vi "Path (SubVI).vi"(1 "File Name":string, 2 "Directory Name":string, 3 "Current VI Name (Case Sensitive)":string, 4 "Current VI Path":path) -> (0 "Path":path)   [LabVIEW 2015]
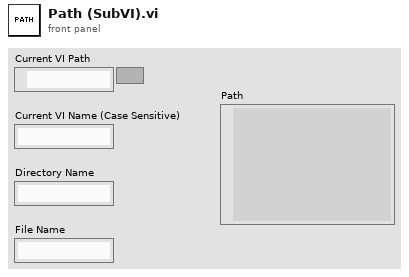
[diagram p1: front panel]
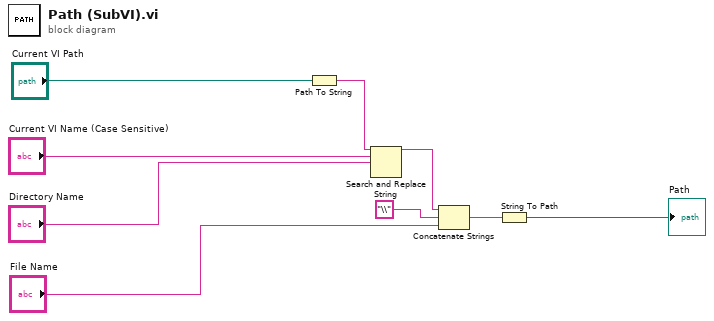
[diagram p0: block diagram]
diagram:
  n1 = Path To String(path="Current VI Path") -> (string=w8:string)
  n2 = Search and Replace String(input string=w8, search string="Current VI Name (Case Sensitive)", replace string="Directory Name") -> (result string=w5:string)  [unwired: 5 in, 3 out]
  n3 = Concatenate Strings(w5, "\\" ("string"), "File Name") -> (w4:string)
  n4 = String To Path(string=w4) -> (path=→"Path":path)
